vi "TimerRun.vi"() -> ()   [LabVIEW 2016]
panel:
  out "Running?":bool
  in  "Timer exec(sec)":u32
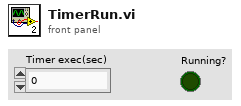
[diagram p1: front panel]
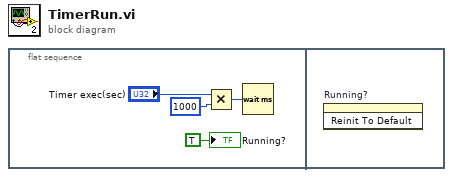
[diagram p0: block diagram]
diagram:
  n1 = flat-sequence {
    frame #0 {
      n2 = Multiply(x="Timer exec(sec)", y=u32 1000) -> (x*y=w2:u32)
      n3 = Wait (ms)(milliseconds to wait=w2) -> ()  [unwired: 1 out]
      "Running?" <- TRUE ("Running?")
    }
    frame #1 {
      n4 = invoke on="Running?" class="Bool (strict)" method="Reinit To Default"() -> ()  [unwired: 3 in, 3 out]
    }
  }
